vi "Get Sync Refnums.vi"(8 "error in (no error)":errorcluster) -> (0 "error out":errorcluster, 2 "Event Sync":T1, 3 "Module Sync":T1)   [LabVIEW 2018, in "Cage Diagram.lvlib"]
doc: "Create or obtain the sync refnums used to synchronize event generation and event registration between the module and its caller(s).\n_____\nBased on Delacor QMH Project Template 4.2.1.64."
uses:
  Cage Diagram.lvlib
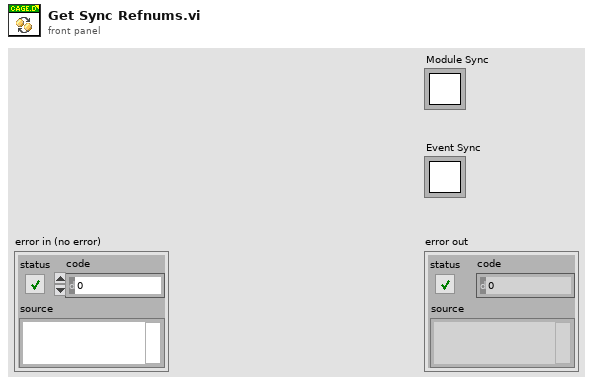
[diagram p1: front panel]
types:
  T1 = typedef "Rendezvous RefNum" = refnum<k1>
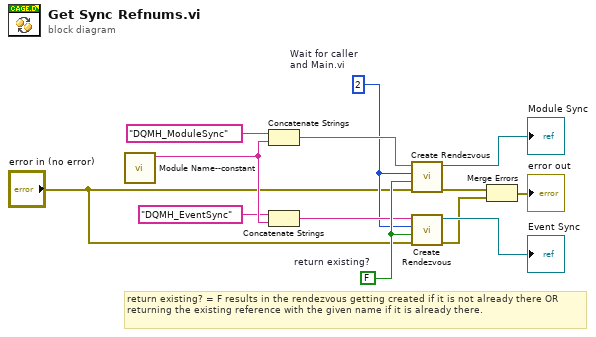
[diagram p0: block diagram]
diagram:
  w7 = FALSE  # return existing?
  w2 = 2  # Wait for caller and Main.vi
  # "return existing? = F results in the rendezvous getting created if it is not already there OR\nreturning the existing reference with the given name if it is already there."
  n1 = call "Module Name--constant.vi"() -> ("Module Name"=w13:string)  [unwired: 11 in]
  n2 = Concatenate Strings("DQMH_ModuleSync" ("name (unnamed)"), w13) -> (w4:string)
  n3 = Concatenate Strings("DQMH_EventSync" ("name (unnamed)"), w13) -> (w3:string)
  n4 = call <vilib>:"Create Rendezvous.vi"("error in (no error)"="error in (no error)", "return existing (F)"=w7, "size (2)"=w2, "name (unnamed)"=w4) -> ("error out"=w9:errorcluster, "rendezvous"=→"Module Sync":T1)  [unwired: 1 in, 1 out]
  n5 = call <vilib>:"Create Rendezvous.vi"("error in (no error)"="error in (no error)", "return existing (F)"=w7, "size (2)"=w2, "name (unnamed)"=w3) -> ("error out"=w8:errorcluster, "rendezvous"=→"Event Sync":T1)  [unwired: 1 in, 1 out]
  n6 = Merge Errors(w9, w8) -> (→"error out":errorcluster)
